vi "PythonCloseTCP.vi"(0 "connection in":refnum<k5>, 7 "run_tcp":bool, 9 "error in":errorcluster) -> (4 "error out":errorcluster)   [LabVIEW 2014]
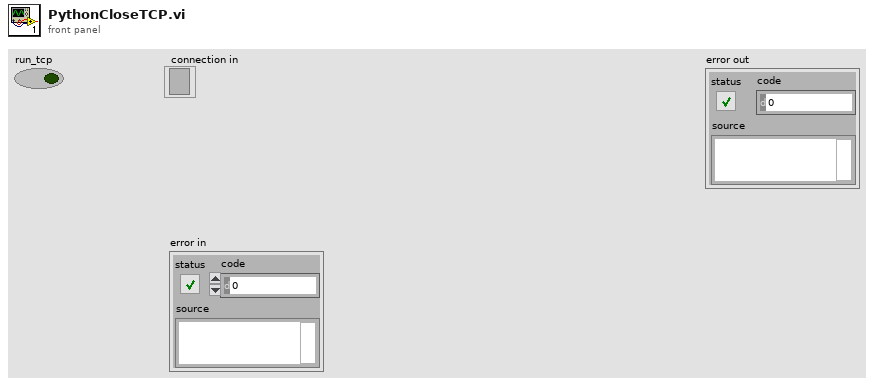
[diagram p1: front panel]
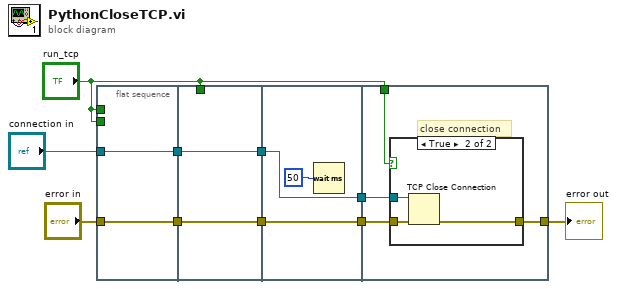
[diagram p0: block diagram]
diagram:
  n1 = flat-sequence {
    tunnel: "error in" -> [w11]
    tunnel: "run_tcp" -> [_]
    tunnel: [w12] -> w8
    tunnel: [w11] -> w7
    tunnel: "connection in" -> [w12]
    tunnel: "run_tcp" -> [_]
    tunnel: [w14] -> w6
    tunnel: w8 -> [w14]
    tunnel: [w13] -> w4
    tunnel: w7 -> [w13]
    tunnel: "run_tcp" -> [_]
    tunnel: w6 -> [w17]
    tunnel: [w17] -> w5
    tunnel: w4 -> [w16]
    tunnel: [w16] -> w3
    tunnel: "run_tcp" -> [w21]
    tunnel: w5 -> [w20]
    tunnel: w3 -> [w19]
    tunnel: [w18] -> w2
    frame #0 {
    }
    frame #1 {
    }
    frame #2 {
      n2 = Wait (ms)(milliseconds to wait=u32 50) -> ()  [unwired: 1 out]
    }
    frame #3 {
      # "close connection"
      n3 = case shown="True" w21 {
        tunnel: w20 -> [_ w25]
        tunnel: w19 -> [w22 w24]
        tunnel: [w22 w23] -> w18
        frame False {
        }
        frame True {
          n4 = TCP Close Connection(connection ID=w25, error in (no error)=w24) -> (error out=w23:errorcluster)  [unwired: 1 in, 1 out]
        }
      }
    }
  }
  "error out" <- w2
